vi "SCMP - Externally Triggered Image Acquisition - v2.vi"(0 "FPS":dbl=10.0 format="%.1g", 1 "LCVR Voltages":dbl[][](array[numeric]), 5 "Modulation Cycles":i32=1 min=1 max=30 step=1, 7 "Save to FITS?":bool=TRUE, 9 "Headers In":T12[](array[typedef])=[{"Wavelength (nm)"=530.15, "Exposure (s)"=0.05, "Tuning Delay (ms)"=1000.0, "Beam Type (-1/1)"=1.0, "Tuning Voltages"=[1.111, 2.222, 3.333, 4.444], "Observer"="observer", "Light Shapping Diffuser"=enum."In Beam", "Comment"="", "Data Type"=9, "Mod Cycles"=0, "SCD Calibration Optics"=enum."1 - Polarizer @0, I+Q", "SCD Emission Line Filter"=enum."1-557.6nm", "Cookbook"="", "COMP-S Calibration Wheel"=enum."Dark", "COMP-S Andover Filter Wheel"=enum."530.3nm/HWB 0.34nm (Fe XIV)", "FOV Rotation (deg)"=66.0, "Objective Lens Position (mm)"=0.0, "Occulter size"=0.0, "Time End"=timestamp(3382374145.421875 s since 1904-01-01), "Acc Exposure (s)"=0.0, "Time Stamp Array"=[], "Camera Serial Number"=[], "Camera Temp"=[], "Camera PI (mm)"=[], "Time Start"=timestamp(3382374145.421875 s since 1904-01-01), "Peripherals"={"ILX controler"=FALSE, "Zone temperatures"=FALSE, "Andor"=FALSE, "Andor 2"=FALSE, "PI Stages"=FALSE, "AISAS mechanisms"=FALSE, "AISAS Mech.lvclass"=refnum, "Zone temp ref"=variant, "FWs"=FALSE}, "FITS paths"=[], "Cameras"=enum."Andor", "load preset cbk"=FALSE, "periodic check count"=0, "COMP-S Calibration Wheel 2"=enum."Dark", "Calib"=enum."Dark", "Abso Aperture"=40.0, "Nominal Aperture"=196.0}] {"Nominal Aperture" format="%.1f"; "Abso Aperture" format="%.1f"; "Camera PI (mm)" format="%_3g"; "Acc Exposure (s)" format="%^.3g"; "Occulter size" format="%.2f"; "Objective Lens Position (mm)" min=70.0 max=152.0 format="%.2f"; "FOV Rotation (deg)" format="%.1f"; "Data Type" items=["LIVE", "DARK", "FLAT", "CALI", "OBSE", "ABSO", "AURE", "TARG", "OBJE", "HOLE", "OREX", "THRO", "CHIP"]; "Exposure (s)" format="%^.3g"; "Wavelength (nm)" format="%_6g"}, 11 "error in":errorcluster, 12 "Andor Neo":T13[](array[typedef]) {"Exposure (s)" format="%^.3g"; "Time at Synch" format="%<%H:%M:%S>T"; "Interframe Time" format="%#_3g"; "Frame Readout Time" format="%_3g"; "Row Readout Time" format="%_3g"}) -> (3 "FITS Path Out":path, 6 "Image":u32[][](array[numeric]), 8 "Image Cam2":u32[][](graph), 10 "Headers Out":T2[](array[typedef]) {"Nominal Aperture" format="%.1f"; "Abso Aperture" format="%.1f"; "Camera PI (mm)" format="%_3g"; "Acc Exposure (s)" format="%^.3g"; "Occulter size" format="%.2f"; "Objective Lens Position (mm)" min=70.0 max=152.0 format="%.2f"; "FOV Rotation (deg)" format="%.1f"; "Exposure (s)" format="%^.3g"; "Wavelength (nm)" format="%_6g"}, 13 "FITS Path Out 2":path, 14 "Break":bool, 15 "error out":errorcluster)   [LabVIEW 2014]
doc: "The LL Sequence VI acquires a sequence of images and displays them in an array of image controls using the low-level acquisition VIs. A sequence is appropriate for applications that process multiple images. You can configure a sequence to acquire every frame or to skip a variable number of frames between each image.\n\nTop Level Code Overview\n1) Initialize Camera (Global Shutter, High Well, Low Noise, exposure time, etc.)\n2) Create a buffer set equal in size to the # of trigger pulses (e.g. 100) which is the same as the # of expected images \n3) Start the camera acquisition THEN start the DAQmx task (use merge error cluster to gurantee this)"
uses:
  Camera/Andor Neo Info.ctl
  <vilib>/DAQmx/configure/timing.llb/DAQmx Timing (Use Waveform).vi
  <vilib>/DAQmx/create/channels.llb/DAQmx Create Channel (AO-Voltage-Basic).vi
  <vilib>/DAQmx/write.llb/DAQmx Write (Analog 1D Wfm NChan NSamp).vi
  <vilib>/Waveform/WDTOps.llb/WDT Waveform Duration DBL.vi
  Controls/beaning.ctl
  Controls/SCD - Calibration Optics Filter Wheel.ctl
  AISAS/Controls/Diffuser.ctl
  Controls/SCD - FITS Cluster.ctl
  Controls/SCD - EDT - Emission Line Filter Wheel.ctl
  Controls/CoMP-S Controls/Polarization Optics Filter Wheel.ctl
  Controls/CoMP-S Controls/Emission Line Filter Wheel.ctl
  AISAS/Controls/focus.ctl
  AISAS/Mech/AISAS Mech.lvclass
  Controls/peripherals.ctl
  Controls/Cameras select.ctl
  Controls/FITS Data type.ctl
panel:
  out "mod cycles *4":i32=1
  out "error dequeue":errorcluster
  out "error dequeue 2":errorcluster
  in  "count 2":i32
  in  "Tab Control":T1(tab)
  in  "user break":bool
  out "Image Cam1 Zoom":u32[][](graph)
  out "Image Cam1":u32[][](graph)
  out "# images to acquire":i32
  out "Image Acquisition Started":bool
  out "PixelData [U16]":u16[](array[numeric])
  out "ByteData [U8]":u8[](array[numeric])
  in  "image pointers":u64[](array[numeric])
  in  "imageNo":i32
  in  "count":i32
  out "Acquisition Estimate (s)":dbl format="%0.2f"
  out "# wavelengths":i32=1
  out "Exposure Get (s)":dbl=0.09 format="%_3p"
  out "Image Acq (s)":dbl(slide)=4151.832132564842
  out "# elements in queue":i32
  out "Image Cam":u32[][](graph)
  out "# buffer":i32
  in  "image pointers 2":u64[](array[numeric])
  in  "imageNo 2":i32
  out "# elements in queue 2":i32
  out "# buffer 2":i32
  out "Time Start":timestamp=timestamp(3382374145.421875 s since 1904-01-01) format="%<%H:%M:%S%3u\n%x>T"
  out "Time stamp arr":timestamp[](array[timestamp]) format="%<%H:%M:%S%3u>T"
  out "COMP Waveforms":waveform(dbl)[](graph)
  out "SCD Waveforms":waveform(dbl)[](graph)
  out "Time stamp arr 2":timestamp[](array[timestamp]) format="%<%H:%M:%S%3u>T"
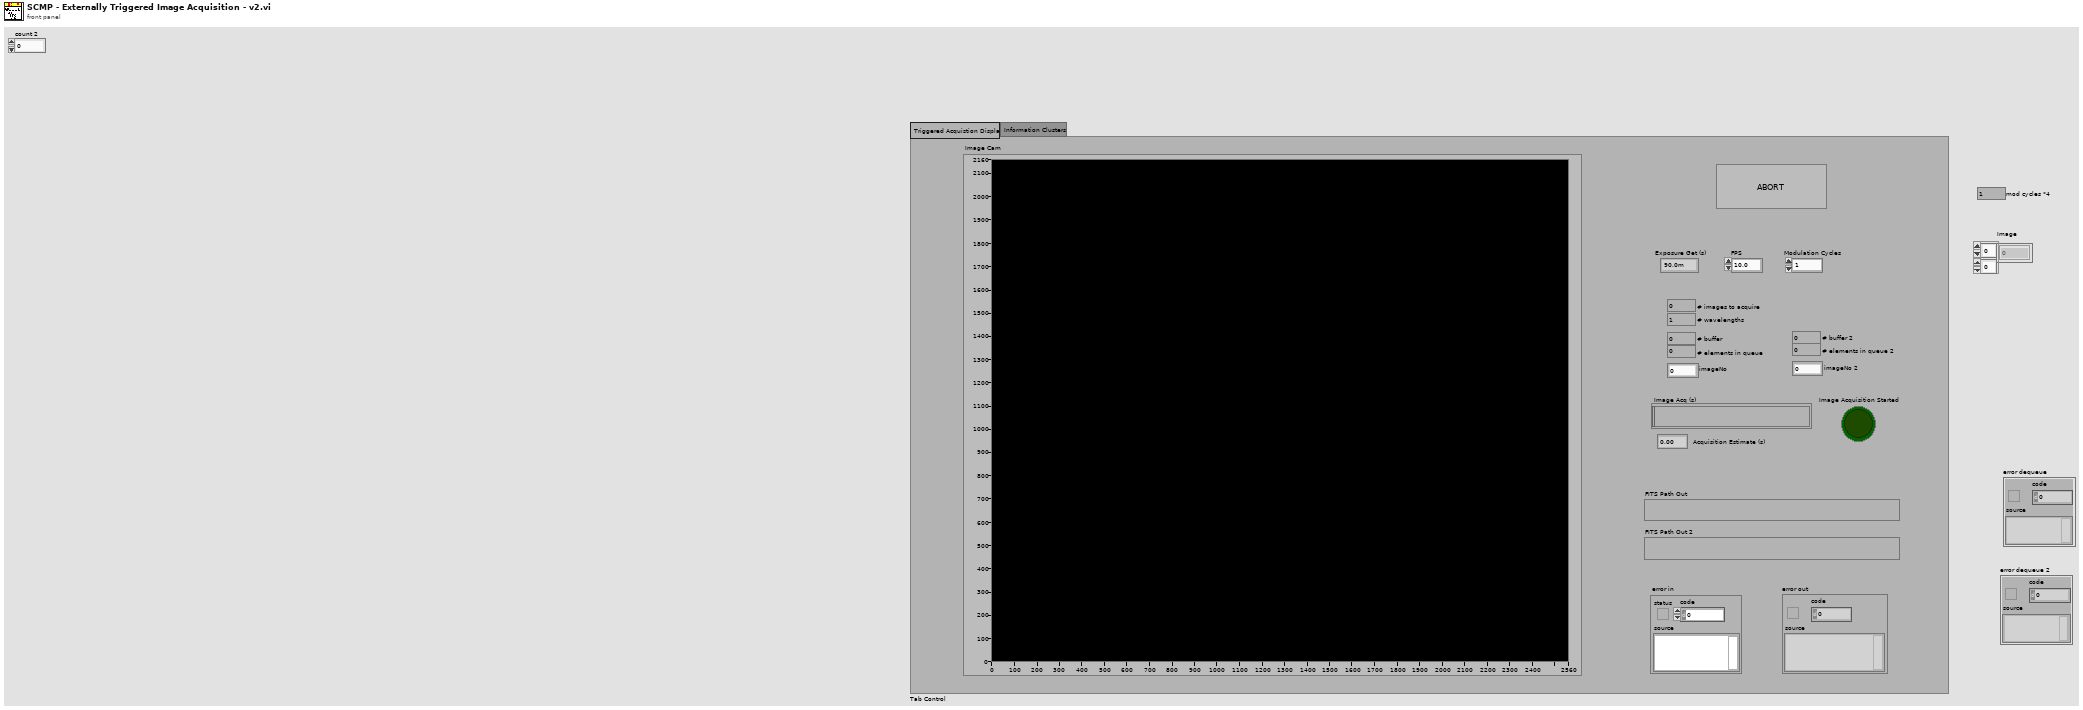
[diagram p1: front panel]
types:
  T1 = enum32{"Triggered Acquistion Display", "Information Clusters"}
  T2 = typedef "SCD - FITS Cluster.ctl" = cluster{"Wavelength (nm)":dbl, "Exposure (s)":dbl, "Tuning Delay (ms)":dbl, "Beam Type (-1/1)":dbl, "Tuning Voltages":dbl[], "Observer":string, "Light Shapping Diffuser":T3, "Comment":string, "Data Type":T4, "Mod Cycles":u16, "SCD Calibration Optics":T5, "SCD Emission Line Filter":T6, "Cookbook":string, "COMP-S Calibration Wheel":T7, "COMP-S Andover Filter Wheel":T8, "FOV Rotation (deg)":dbl, "Objective Lens Position (mm)":T9, "Occulter size":dbl, "Time End":timestamp, "Acc Exposure (s)":dbl, "Time Stamp Array":timestamp[], "Camera Serial Number":string[], "Camera Temp":dbl[], "Camera PI (mm)":dbl[], "Time Start":timestamp, "Peripherals":T10, "FITS paths":path[], "Cameras":T11, "load preset cbk":bool, "periodic check count":i32, "COMP-S Calibration Wheel 2":T7, "Calib":enum16{"Dark", "Flat"}, "Abso Aperture":dbl, "Nominal Aperture":dbl, "Pointer IP":string}
  T3 = typedef "Diffuser.ctl" = enum16{"Out of Beam", "In Beam"}
  T4 = typedef "FITS Data type.ctl" = enum16{"LIVE", "DARK", "FLAT", "CALI", "OBSE", "ABSO", "AURE", "TARG", "OBJE", "HOLE", "OREX", "THRO", "CHIP"}
  T5 = typedef "SCD - Calibration Optics Filter Wheel.ctl" = enum16{"1 - Polarizer @0, I+Q", "2 - Polarizer @90, I-Q", "3 - Polarizer @45, I+U", "4 - Polarizer @135, I-U", "5 - Polarizer @0, Retarder @45, I+V", "6 - Polarizer @0, Retarder @135, I-V", "7 - Dark", "8 - Clear", "9 - N/A"}
  T6 = typedef "SCD - EDT - Emission Line Filter Wheel.ctl" = enum16{"1-557.6nm", "2-587.6nm", "3-589.6nm", "4-630.2nm", "5-656.4nm", "6-849.8nm", "7-854.2nm", "8-866.2nm", "9-1083.0nm"}
  T7 = typedef "Polarization Optics Filter Wheel.ctl" = enum16{"Dark", "Clear", "Exchange Lens", "Polarizer @0, I+Q", "Polarizer @90, I-Q", "Polarizer @45, I+U", "Polarizer @135, I-U", "Polarizer @0, Retarder @45, I+V", "Polarizer @0, Retarder @135, I-V"}
  T8 = typedef "Emission Line Filter Wheel.ctl" = enum16{"530.3nm/HWB 0.34nm (Fe XIV)", "587.6nm/HBW 0.44nm (He I D3)", "637.5nm/HBW 0.53nm (Fe X)", "656.3nm/HBW 0.57nm (H-Alpha)", "789.2nm/HBW 0.85nm (Fe XI)", "854.2nm/HBW 1.01nm (Ca I)", "1074.7nm/HBW 2.34nm (Fe XIII)", "1079.8nm/HBW 1.64nm (Fe XIII)", "1083.0nm/HBW 1.66nm (He I)"}
  T9 = typedef "focus.ctl" = dbl
  T10 = typedef "peripherals.ctl" = cluster{"ILX controler":bool, "Zone temperatures":bool, "Andor":bool, "Andor 2":bool, "PI Stages":bool, "AISAS mechanisms":bool, "AISAS Mech.lvclass":refnum<class "AISAS Mech.lvclass">, "Zone temp ref":variant, "FWs":bool}
  T11 = typedef "Cameras select.ctl" = enum16{"Andor", "GDR"}
  T12 = typedef "SCD - FITS Cluster.ctl" = cluster{"Wavelength (nm)":dbl, "Exposure (s)":dbl, "Tuning Delay (ms)":dbl, "Beam Type (-1/1)":dbl, "Tuning Voltages":dbl[], "Observer":string, "Light Shapping Diffuser":T3, "Comment":string, "Data Type":u16, "Mod Cycles":u16, "SCD Calibration Optics":T5, "SCD Emission Line Filter":T6, "Cookbook":string, "COMP-S Calibration Wheel":T7, "COMP-S Andover Filter Wheel":T8, "FOV Rotation (deg)":dbl, "Objective Lens Position (mm)":T9, "Occulter size":dbl, "Time End":timestamp, "Acc Exposure (s)":dbl, "Time Stamp Array":timestamp[], "Camera Serial Number":string[], "Camera Temp":dbl[], "Camera PI (mm)":dbl[], "Time Start":timestamp, "Peripherals":T10, "FITS paths":path[], "Cameras":T11, "load preset cbk":bool, "periodic check count":i32, "COMP-S Calibration Wheel 2":T7, "Calib":enum16{"Dark", "Flat"}, "Abso Aperture":dbl, "Nominal Aperture":dbl}
  T13 = typedef "Andor Neo Info.ctl" = cluster{"Handle":i32, "Pixel Encoding":string, "AOI Width":i32, "AOI Height":i32, "AOI Stride":i32, "Row Readout Time":dbl, "Frame Readout Time":dbl, "Interframe Time":dbl, "Semaphore":T14, "SerialNumber":string, "Camera Model":string, "Controller ID":string, "Firmware Version":string, "Shutter":string, "BDiv":u8, "Time at Synch":timestamp, "Idx":i32, "PreAmp":string, "Binning":T15, "PixelReadoutRate":string, "Exposure (s)":dbl, "Image Bytes":i64, "Image Pixels":i64, "SpuriousNoiseFilter":bool, "Overlap":bool, "CycleMode":string}
  T14 = typedef "Semaphore RefNum" = refnum<k1>
  T15 = typedef "beaning.ctl" = enum16{"1x1", "2x2", "3x3", "4x4", "8x8"}
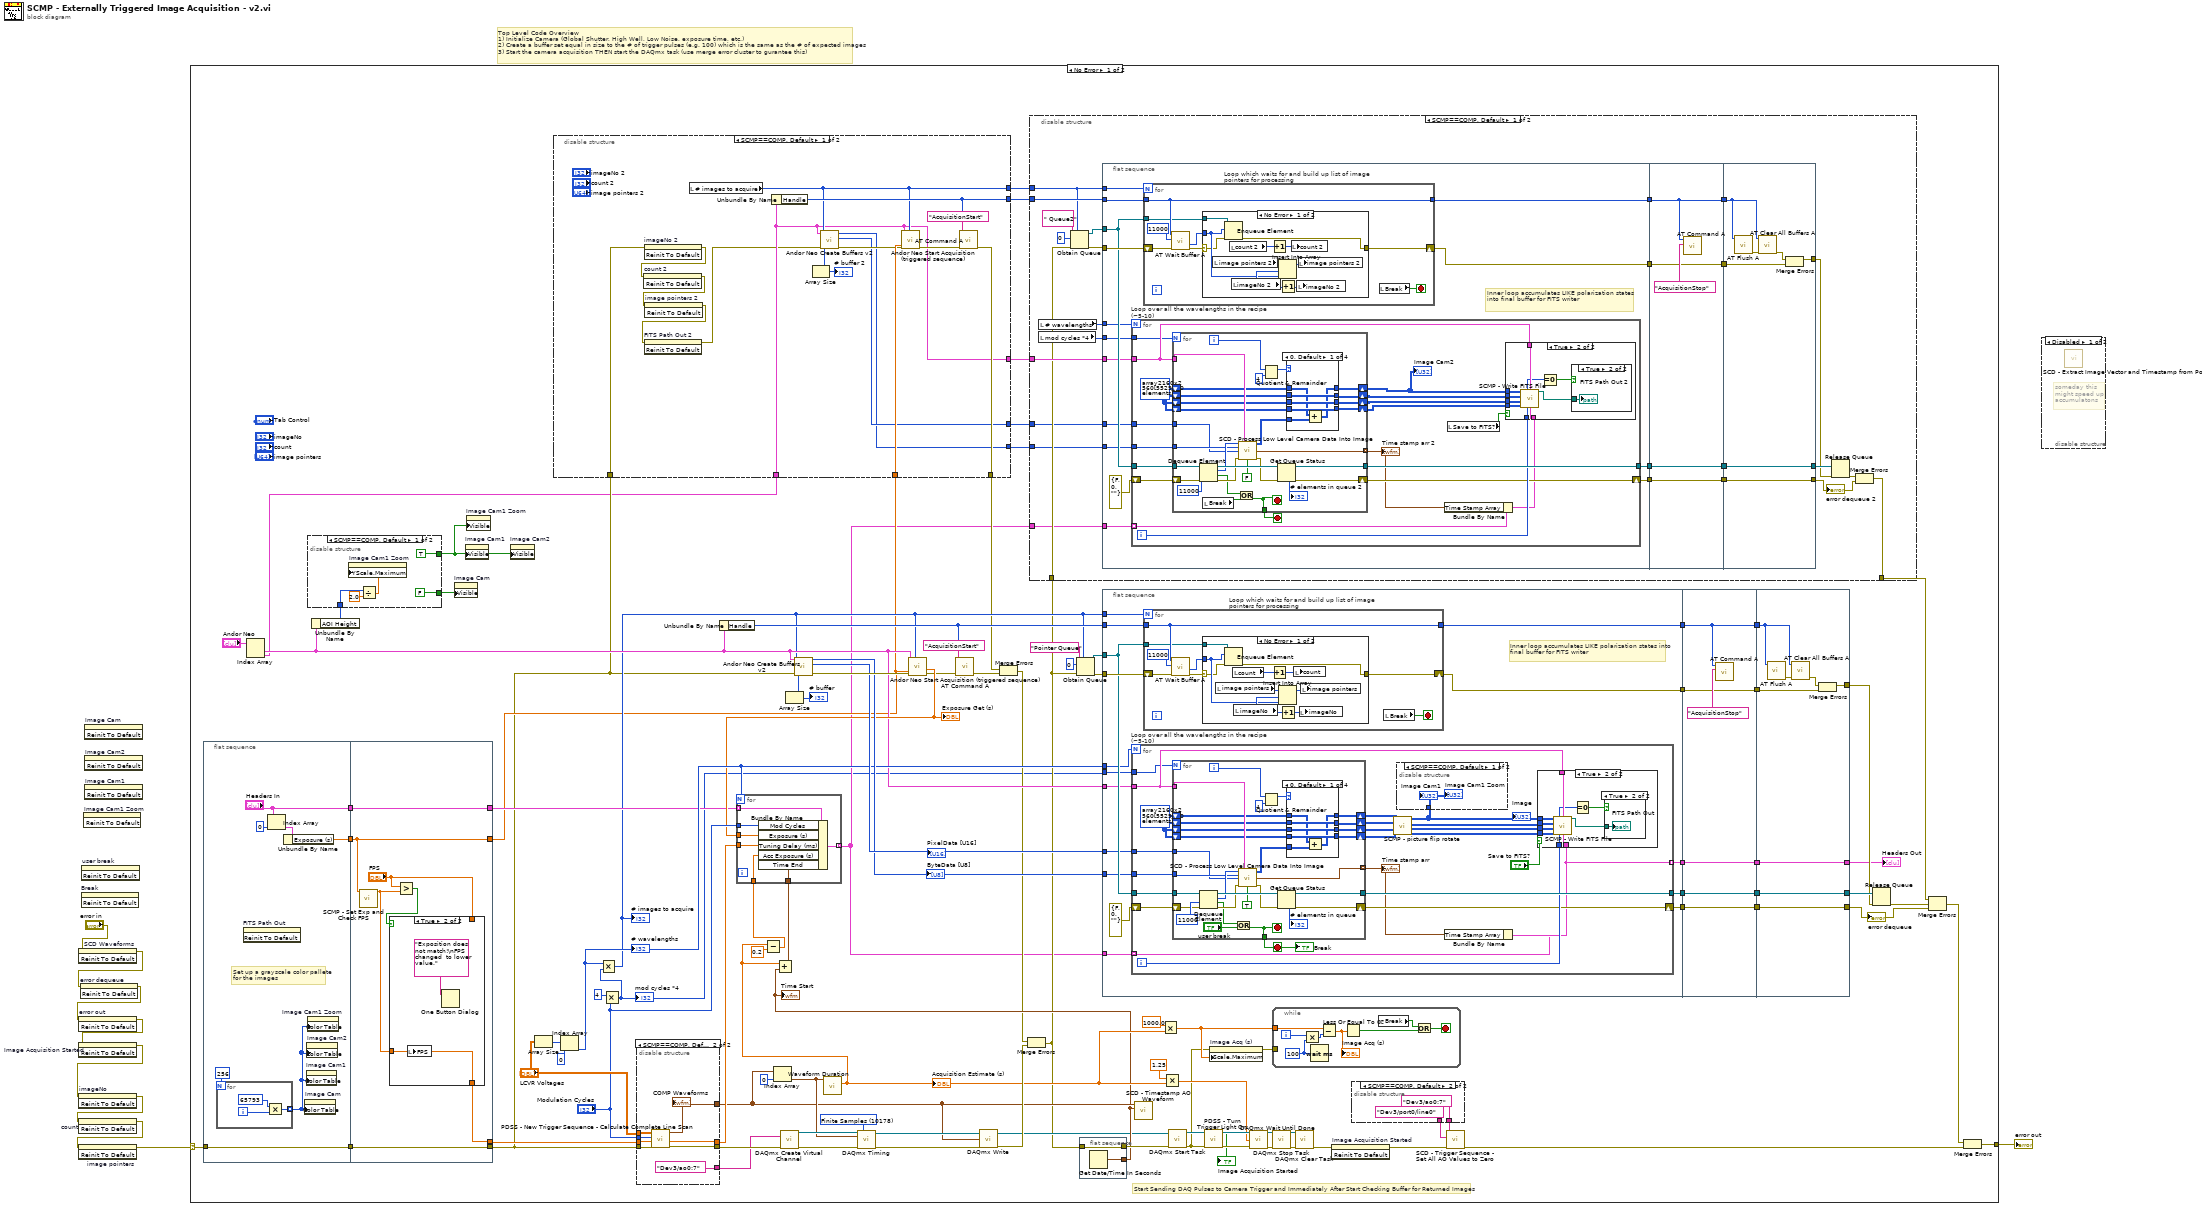
[diagram p0: block diagram]
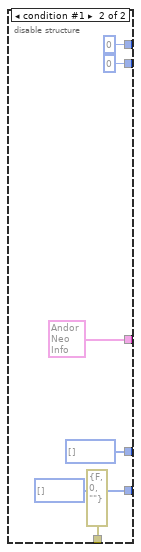
[diagram p3: hidden frame]
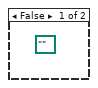
[diagram p4: hidden frame]
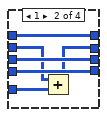
[diagram p6: hidden frame]
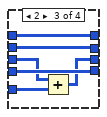
[diagram p7: hidden frame]
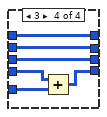
[diagram p8: hidden frame]
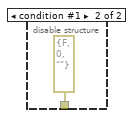
[diagram p10: hidden frame]
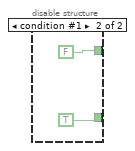
[diagram p12: hidden frame]
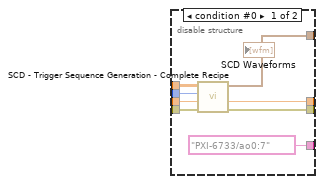
[diagram p13: hidden frame]
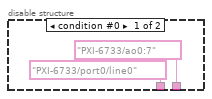
[diagram p14: hidden frame]
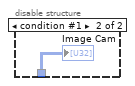
[diagram p15: hidden frame]
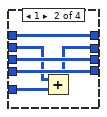
[diagram p18: hidden frame]
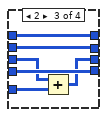
[diagram p19: hidden frame]
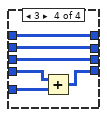
[diagram p20: hidden frame]
diagram:
  # "Top Level Code Overview\n1) Initialize Camera (Global Shutter, High Well, Low Noise, exposure time, etc.)\n2) Create a buffer set equal in size to the # of trigger pulses (e.g. 100) which is the same as the # of expected images \n3) Start the camera acquisition THEN start the DAQmx task (use merge error cluster to gurantee this)"
  n1 = invoke on="SCD Waveforms" class="WFGraph (strict)" method="Reinit To Default"(error in="error in") -> (error out=w3:errorcluster)  [unwired: 2 in, 2 out]
  n2 = invoke on="error dequeue" class="Clust (strict)" method="Reinit To Default"(error in=w3) -> (error out=w2:errorcluster)  [unwired: 2 in, 2 out]
  n3 = invoke on="error out" class="Clust (strict)" method="Reinit To Default"(error in=w2) -> (error out=w8:errorcluster)  [unwired: 2 in, 2 out]
  n4 = invoke on="Image Acquisition Started" class="Bool (strict)" method="Reinit To Default"(error in=w8) -> (error out=w4:errorcluster)  [unwired: 2 in, 2 out]
  n5 = invoke on="imageNo" class="DigNum (strict)" method="Reinit To Default"(error in=w4) -> (error out=w7:errorcluster)  [unwired: 2 in, 2 out]
  n6 = invoke on="count" class="DigNum (strict)" method="Reinit To Default"(error in=w7) -> (error out=w6:errorcluster)  [unwired: 2 in, 2 out]
  n7 = invoke on="image pointers" class="Arr (strict)" method="Reinit To Default"(error in=w6) -> (error out=w5:errorcluster)  [unwired: 2 in, 2 out]
  n8 = invoke on="Break" class="Bool (strict)" method="Reinit To Default"() -> ()  [unwired: 3 in, 3 out]
  n9 = invoke on="user break" class="Bool (strict)" method="Reinit To Default"() -> ()  [unwired: 3 in, 3 out]
  n10 = invoke on="Image Cam1 Zoom" class="IntGraph (strict)" method="Reinit To Default"() -> ()  [unwired: 3 in, 3 out]
  n11 = invoke on="Image Cam" class="IntGraph (strict)" method="Reinit To Default"() -> ()  [unwired: 3 in, 3 out]
  n12 = invoke on="Image Cam2" class="IntGraph (strict)" method="Reinit To Default"() -> ()  [unwired: 3 in, 3 out]
  n13 = invoke on="Image Cam1" class="IntGraph (strict)" method="Reinit To Default"() -> ()  [unwired: 3 in, 3 out]
  n14 = case shown="No Error" w5 {
    selector: w5 -> [w45 w491]
    tunnel: [w82 w491] -> w9
    frame No Error {
      w109 = 10178 items=["Finite Samples"=10178, "Continuous Samples"=10123] ("sample mode")
      # "Start Sending DAQ Pulses to Camera Trigger and Immediately After Start Checking Buffer for Returned Images"
      n15 = flat-sequence {
        tunnel: w45 -> [w294]
        tunnel: [w294] -> w37
        tunnel: ["Headers In"] -> w35
        tunnel: [w289] -> w34
        tunnel: [w305] -> w13
        tunnel: w37 -> [w305]
        tunnel: [w304] -> w36
        tunnel: w35 -> [w304]
        tunnel: [w299] -> w23
        tunnel: w34 -> [w299]
        tunnel: [w302] -> w33
        frame #0 {
          # "Set up a grayscale color pallete for the images"
          n16 = for {
            N: 256 -> [_]
            tunnel: [w297] -> w293 mode=indexing
            i -> [w298]
            n17 = Multiply(x=65793, y=w298) -> (x*y=w297:i32)
          }
          n18 = invoke on="FITS Path Out" class="Path" method="Reinit To Default"() -> ()  [unwired: 3 in, 3 out]
          n19 = Index Array(array="Headers In", index=0) -> (element=w291:T12)
          n20 = Unbundle By Name(w291) -> ("Exposure (s)"=w289:dbl)
          n21 = property on="Image Cam" class="IntGraph (strict)"("Color Table"=w293) -> ()  [unwired: 2 in, 2 out]
          n22 = property on="Image Cam1" class="IntGraph (strict)"("Color Table"=w293) -> ()  [unwired: 2 in, 2 out]
          n23 = property on="Image Cam2" class="IntGraph (strict)"("Color Table"=w293) -> ()  [unwired: 2 in, 2 out]
          n24 = property on="Image Cam1 Zoom" class="IntGraph (strict)"("Color Table"=w293) -> ()  [unwired: 2 in, 2 out]
        }
        frame #1 {
          n25 = call "SCMP - Set Exp and Check FPS.vi"("Exposure [s]"=w299) -> ("FPS"=w300:dbl)  [unwired: 9 in, 1 out]
          n26 = Greater?(x="FPS", y=w300) -> (0:w303:bool)
          n27 = case shown="True" w303 {
            tunnel: [w306 w307] -> w302
            tunnel: "FPS" -> [w306 _]
            tunnel: w300 -> [_ w307]
            frame False {
            }
            frame True {
              n28 = local write "FPS"(w307) -> ()
              n29 = One Button Dialog(message="Exposition does not match!\nFPS changed  to lower value.") -> ()  [unwired: 1 in, 1 out]
            }
          }
        }
      }
      n30 = Index Array(array="Andor Neo") -> (element #1=w27:T13, element #2=w10:T13)  [unwired: 2 in]
      n31 = Unbundle By Name(w27) -> ("AOI Height"=w54:i32)
      n32 = disable-structure shown="SCMP==COMP, Default" {
        disable-tunnel: w54 -> [w312 _]
        disable-tunnel: [TRUE ("Visible") FALSE ("Visible")] -> w46
        disable-tunnel: [FALSE ("Visible") TRUE ("Visible")] -> w53
        frame condition #0 (active) {
          n33 = Divide(x=w312, y=2.0) -> (x/y=w313:dbl)
          n34 = property on="Image Cam1 Zoom" class="IntGraph (strict)"("YScale.Maximum"=w313) -> ()  [unwired: 2 in, 2 out]
        }
        frame condition #1 {
        }
      }
      n35 = property on="Image Cam" class="IntGraph (strict)"("Visible"=w53) -> ()  [unwired: 2 in, 2 out]
      n36 = property on="Image Cam1" class="IntGraph (strict)"("Visible"=w46) -> ()  [unwired: 2 in, 2 out]
      n37 = property on="Image Cam1 Zoom" class="IntGraph (strict)"("Visible"=w46) -> ()  [unwired: 2 in, 2 out]
      n38 = property on="Image Cam2" class="IntGraph (strict)"("Visible"=w46) -> ()  [unwired: 2 in, 2 out]
      n39 = Array Size(array="LCVR Voltages") -> (size(s)=w92:i32[])
      n40 = disable-structure shown="SCMP==COMP, Default" {
        disable-tunnel: w23 -> [w126 _]
        disable-tunnel: [w125 errorcluster {"status"=FALSE, "code"=0, "source"=""} ("error out")] -> w20
        disable-tunnel: [w119 0 ("Handle")] -> w17
        disable-tunnel: [w118 i64[] [] ("PixelData")] -> w16
        disable-tunnel: [w117 u8[] [] ("ByteData")] -> w15
        disable-tunnel: [w116 0 ("# images to acquire")] -> w14
        disable-tunnel: w13 -> [w112 _]
        disable-tunnel: [w115 T13 {"Handle"=0, "Pixel Encoding"="", "AOI Width"=0, "AOI Height"=0, "AOI Stride"=0, "Row Readout Time"=0.0, "Frame Readout Time"=0.0, "Interframe Time"=0.0, "Semaphore"=refnum, "SerialNumber"="", "Camera Model"="", "Controller ID"="", "Firmware Version"="", "Shutter"="Global", "BDiv"=1, "Time at Synch"=timestamp(3029526000.379448 s since 1904-01-01), "Idx"=0, "PreAmp"="", "Binning"=enum."1x1", "PixelReadoutRate"="", "Exposure (s)"=0.05, "Image Bytes"=0, "Image Pixels"=0, "SpuriousNoiseFilter"=FALSE, "Overlap"=FALSE, "CycleMode"=""} ("Neo Info")] -> w11
        disable-tunnel: w10 -> [w115 _]
        frame condition #0 (active) {
          n41 = invoke on="imageNo 2" class="DigNum (strict)" method="Reinit To Default"(error in=w112) -> (error out=w114:errorcluster)  [unwired: 2 in, 2 out]
          n42 = invoke on="count 2" class="DigNum (strict)" method="Reinit To Default"(error in=w114) -> (error out=w113:errorcluster)  [unwired: 2 in, 2 out]
          n43 = invoke on="image pointers 2" class="Arr (strict)" method="Reinit To Default"(error in=w113) -> (error out=w111:errorcluster)  [unwired: 2 in, 2 out]
          n44 = invoke on="FITS Path Out 2" class="Path" method="Reinit To Default"(error in=w111) -> (error out=w110:errorcluster)  [unwired: 2 in, 2 out]
          n45 = local read "# images to acquire"() -> (w116:i32)
          n46 = Unbundle By Name(w115) -> ("Handle"=w119:i32)
          n47 = call "Andor Neo Create Buffers v2.vi"("error in"=w110, "Number of Images"=w116, "Camera Info"=w115) -> ("error out"=w123:errorcluster, "PixelData"=w118:i64[], "ByteData"=w117:u8[], "# of Andor buffers"=w121:i32)  [unwired: 4 in, 1 out]
          n48 = Array Size(array=w121) -> (size(s)=→"# buffer 2":i32)
          n49 = call "Andor Neo Start Acquisition (triggered sequence).vi"("Exposure Set (s)"=w126, "error in"=w123, "Frames"=w116, "Camera Info"=w115) -> ("error out"=w122:errorcluster)  [unwired: 6 in, 1 out]
          n50 = call <userlib>:"AT Command A.vi"("error in (no error)"=w122, "Feature"="AcquisitionStart" ("Command"), "Handle"=w119) -> ("error out"=w125:errorcluster)  [unwired: 7 in, 1 out]
        }
        frame condition #1 {
        }
      }
      n51 = Index Array(array=w92, index=0) -> (element=w55:i32)
      "# wavelengths" <- w55
      n52 = Multiply(x=4 ("value"), y="Modulation Cycles") -> (x*y=w12:i32)
      "mod cycles *4" <- w12
      n53 = Multiply(x=w55, y=w12) -> (x*y=w24:i32)
      "# images to acquire" <- w24
      n54 = disable-structure shown="SCMP==COMP, Default" {
        disable-tunnel: [w323 w327] -> w100
        disable-tunnel: "LCVR Voltages" -> [w322 w331]
        disable-tunnel: [w317 w325] -> w60
        disable-tunnel: w33 -> [w321 w329]
        disable-tunnel: w13 -> [w320 w328]
        disable-tunnel: [w319 w326] -> w63
        disable-tunnel: "Modulation Cycles" -> [w318 w330]
        disable-tunnel: [tag "PXI-6733/ao0:7" ("physical channels") tag "Dev3/ao0:7" ("physical channels")] -> w31
        frame condition #0 {
          n55 = call "SCD - Trigger Sequence Generation - Complete Recipe.vi"("error in"=w320, "FPS"=w321, "Modulation Cycles\nAt Each Wavelength"=w318, "LCVR Voltages"=w322) -> ("error out"=w323:errorcluster, "LCVR Relaxtion Time"=w319:dbl, "SCD Waveforms (Graph)"=w317:waveform(dbl)[])  [unwired: 5 in]
          "SCD Waveforms" <- w317
        }
        frame condition #1 (active) {
          n56 = call "PDSS - New Trigger Sequence - Calculate Complete Line Scan.vi"("error in"=w328, "FPS"=w329, "Modulation Cycles\nAt Each Wavelength"=w330, "LCVR Voltages"=w331) -> ("error out"=w327:errorcluster, "LCVR Relaxtion Time"=w326:dbl, "AO Graph"=w325:waveform(dbl)[])  [unwired: 5 in]
          "COMP Waveforms" <- w325
        }
      }
      n57 = Unbundle By Name(w27) -> ("Handle"=w26:i32)
      n58 = Index Array(array=w60, index=0) -> (element=w97:waveform(dbl))
      n59 = call-poly <vilib>:"DAQmx Create Virtual Channel.vi"("physical channels"=w31, "error in"=w100) -> ("task out"=w107:refnum<k21>, "error out"=w108:errorcluster)  [unwired: 12 in]
      n60 = call "Andor Neo Create Buffers v2.vi"("error in"=w13, "Number of Images"=w24, "Camera Info"=w27) -> ("error out"=w81:errorcluster, "PixelData"=w77:i64[], "ByteData"=w76:u8[], "# of Andor buffers"=w44:i32)  [unwired: 4 in, 1 out]
      "ByteData [U8]" <- w76
      "PixelData [U16]" <- w77
      n61 = Array Size(array=w44) -> (size(s)=→"# buffer":i32)
      n62 = call-poly <vilib>:"Waveform Duration.vi"("waveform in"=w97) -> ("duration"=w48:dbl)  [unwired: 8 in, 2 out]
      "Acquisition Estimate (s)" <- w48
      n63 = Subtract(x=w48, y=0.2) -> (x-y=w47:dbl)
      n64 = Add(x=w48, y=w32) -> (x+y=w52:timestamp)
      n65 = call-poly <vilib>:"DAQmx Timing.vi"("task/channels in"=w107, "sample mode"=w109, "waveform"=w97, "error in"=w108) -> ("task out"=w98:refnum<k21>, "error out"=w99:errorcluster)  [unwired: 10 in]
      n66 = call "Andor Neo Start Acquisition (triggered sequence).vi"("Exposure Set (s)"=w23, "error in"=w81, "Frames"=w24, "Camera Info"=w27) -> ("error out"=w50:errorcluster, "Exposure Get (s)"=w51:dbl)  [unwired: 6 in]
      "Exposure Get (s)" <- w51
      n67 = for {
        N: w55 -> [_]
        tunnel: [w350] -> w19 mode=indexing
        tunnel: w51 -> [w349]
        tunnel: w36 -> [w348] mode=indexing
        tunnel: w63 -> [w347]
        tunnel: "Modulation Cycles" -> [w346]
        tunnel: w47 -> [w345]
        tunnel: w52 -> [w344]
        n68 = Bundle By Name(cluster=w348, "Mod Cycles"=w346, "Exposure (s)"=w349, "Tuning Delay (ms)"=w347, "Acc Exposure (s)"=w345, "Time End"=w344) -> (w350:T12)
      }
      n69 = call <userlib>:"AT Command A.vi"("error in (no error)"=w50, "Feature"="AcquisitionStart" ("Command"), "Handle"=w26) -> ("error out"=w80:errorcluster)  [unwired: 7 in, 1 out]
      n70 = call-poly <vilib>:"DAQmx Write.vi"("task/channels in"=w98, "data"=w60, "error in"=w99) -> ("task out"=w25:refnum<k21>, "error out"=w84:errorcluster)  [unwired: 10 in, 1 out]
      n71 = Merge Errors(w20, w80) -> (w21:errorcluster)
      n72 = Merge Errors(w21, w84) -> (w22:errorcluster)
      n73 = disable-structure shown="SCMP==COMP, Default" {
        disable-tunnel: w11 -> [w150 _]
        disable-tunnel: w22 -> [w149 _]
        disable-tunnel: w19 -> [w148 _]
        disable-tunnel: [w147 errorcluster {"status"=FALSE, "code"=0, "source"=""} ("error IO")] -> w18
        disable-tunnel: w17 -> [w144 _]
        disable-tunnel: w16 -> [w143 _]
        disable-tunnel: w15 -> [w142 _]
        disable-tunnel: w14 -> [w139 _]
        frame condition #0 (active) {
          n74 = local read "# wavelengths"() -> (w138:i32)
          n75 = local read "mod cycles *4"() -> (w133:i32)
          n76 = Obtain Queue(max queue size (-1, unlimited)=w139, name (unnamed)=" Queue2", element data type=u64 0 ("Output buffer"), error in (no error)=w149) -> (queue out=w141:refnum<queue>, error out=w140:errorcluster)  [unwired: 1 in, 1 out]
          n77 = flat-sequence {
            tunnel: w140 -> [w173]
            tunnel: w144 -> [w172]
            tunnel: [w171] -> w158
            tunnel: [w162] -> w157
            tunnel: w150 -> [w166]
            tunnel: w143 -> [w167]
            tunnel: w142 -> [w169]
            tunnel: w141 -> [w170]
            tunnel: [w168] -> w156
            tunnel: w133 -> [w164]
            tunnel: [w165] -> w155
            tunnel: w139 -> [w161]
            tunnel: w148 -> [w160]
            tunnel: w138 -> [w159]
            tunnel: w158 -> [w277]
            tunnel: w157 -> [w276]
            tunnel: w156 -> [w279]
            tunnel: w155 -> [w278]
            tunnel: [w277] -> w154
            tunnel: [w279] -> w153
            tunnel: [w278] -> w152
            tunnel: [w276] -> w151
            tunnel: [w287] -> w135
            tunnel: [w286] -> w134
            tunnel: w154 -> [w284]
            tunnel: w153 -> [w282]
            tunnel: w152 -> [w287]
            tunnel: w151 -> [w285]
            tunnel: [w282] -> w136
            frame #0 {
              # "Inner loop accumulates LIKE polarization states into final buffer for FITS writer"
              n78 = for "Loop over all the wavelengths in the recipe (~5-10)" {
                N: w159 -> [_]
                tunnel: w170 -> [w192]
                tunnel: w169 -> [w191]
                tunnel: [w190] -> w168
                tunnel: w167 -> [w189]
                tunnel: w166 -> [w187]
                tunnel: w164 -> [w186]
                shift-right: [w184] -> w165
                shift-left: errorcluster {"status"=FALSE, "code"=0, "source"=""} ("error out") -> [w183]
                tunnel: w160 -> [w179] mode=indexing
                i -> [w185]
                stop <- w182 stop-if-true
                w188 = u32[][] array2160x2560[5529600 elements] ("2560x2160 Initialized Array")
                n79 = for {
                  N: w186 -> [_]
                  tunnel: w192 -> [w232]
                  tunnel: w191 -> [w229]
                  tunnel: [w215] -> w190
                  tunnel: w189 -> [w228]
                  tunnel: w187 -> [w227]
                  shift-right: [w220] -> w177
                  shift-left: w188 -> [w221]
                  shift-right: [w219] -> w176
                  shift-left: w188 -> [w222]
                  shift-right: [w218] -> w175
                  shift-left: w188 -> [w223]
                  shift-right: [w217] -> w174
                  shift-left: w188 -> [w224]
                  shift-right: [w210] -> w184
                  shift-left: w183 -> [w208]
                  tunnel: [w205] -> w182
                  tunnel: [w207] -> w180 mode=indexing
                  i -> [w209]
                  stop <- w205 stop-if-true
                  n80 = Dequeue Element(queue=w232, timeout in ms (-1)=11000, error in (no error)=w208) -> (queue out=w231:refnum<queue>, element=w230:u64, timed out?=w204:bool, error out=w212:errorcluster)
                  n81 = local read "Break"() -> (w203:bool)
                  n82 = Or(x=w204, y=w203) -> (x .or. y?=w205:bool)
                  n83 = call "SCD - Process Low Level Camera Data Into Image.vi"("Pointer In"=w230, "Neo Info"=w227, "ByteData (U8)"=w229, "PixelData (U16)"=w228, "error in (no error)"=w212, "scmp demo pic"=FALSE) -> ("Image (I32)"=w216:u32[][], "Timestamp"=w207:timestamp, "error out"=w211:errorcluster)  [unwired: 7 in]
                  n84 = Quotient & Remainder(x=w209, y=4) -> (x-y*floor(x/y)=w225:i32)  [unwired: 1 out]
                  n85 = Get Queue Status(queue=w231, error in (no error)=w211) -> (queue out=w215:refnum<queue>, error out=w210:errorcluster, # elements in queue=→"# elements in queue 2":i32)  [unwired: 1 in, 5 out]
                  n86 = case shown="0, Default" w225 {
                    tunnel: w224 -> [w236 w243 w249 w252]
                    tunnel: w223 -> [w237 w244 w246 w255]
                    tunnel: w222 -> [w238 w240 w250 w256]
                    tunnel: w221 -> [w234 w241 w247 w253]
                    tunnel: [w233 w241 w247 w253] -> w220
                    tunnel: [w238 w239 w250 w256] -> w219
                    tunnel: [w237 w244 w245 w255] -> w218
                    tunnel: [w236 w243 w249 w251] -> w217
                    tunnel: w216 -> [w235 w242 w248 w254]
                    frame 0, Default {
                      n87 = Add(x=w234, y=w235) -> (x+y=w233:u32[][])
                    }
                    frame 1 {
                      n88 = Add(x=w240, y=w242) -> (x+y=w239:u32[][])
                    }
                    frame 2 {
                      n89 = Add(x=w246, y=w248) -> (x+y=w245:u32[][])
                    }
                    frame 3 {
                      n90 = Add(x=w252, y=w254) -> (x+y=w251:u32[][])
                    }
                  }
                }
                "Time stamp arr 2" <- w180
                "Image Cam2" <- w177
                n91 = Bundle By Name(cluster=w179, "Time Stamp Array"=w180) -> (w181:T12)
                n92 = local read "Save to FITS?"() -> (w178:bool)
                n93 = case shown="True" w178 {
                  tunnel: w176 -> [_ w199]
                  tunnel: w175 -> [_ w200]
                  tunnel: w174 -> [_ w201]
                  tunnel: w181 -> [_ w197]
                  tunnel: w177 -> [_ w198]
                  tunnel: w187 -> [_ w196]
                  tunnel: w185 -> [_ w195]
                  frame False {
                    (unwired) path "" ("FITS Path Out")
                  }
                  frame True {
                    n94 = call "SCMP - Write FITS File.vi"("A"=w198, "FITS Header"=w197, "Neo Info"=w196, "B"=w199, "C"=w200, "D"=w201, "Image #"=w195) -> ("FITS Path Out"=w194:path)  [unwired: 6 in, 2 out]
                    n95 = Equal To 0?(x=w195) -> (x = 0?=w193:bool)
                    n96 = case shown="True" w193 {
                      tunnel: w194 -> [_ w202]
                      frame False {
                      }
                      frame True {
                        "FITS Path Out 2" <- w202
                      }
                    }
                  }
                }
              }
              n97 = for "Loop which waits for and build up list of image pointers for processing" {
                N: w161 -> [_]
                tunnel: w172 -> [w261]
                tunnel: [w261] -> w171
                tunnel: w170 -> [w259]
                shift-right: [w258] -> w162
                shift-left: w173 -> [w263]
                stop <- w257 stop-if-true
                n98 = call <userlib>:"AT Wait Buffer A.vi"("error in (no error)"=w263, "Timeout"=u32 11000, "Handle"=w261) -> ("error out"=w260:errorcluster, "Output buffer"=w262:u64)  [unwired: 5 in, 2 out]
                n99 = case shown="No Error" w260 {
                  selector: w260 -> [w266 w275]
                  tunnel: w262 -> [w268 _]
                  tunnel: [w265 w275] -> w258
                  tunnel: w259 -> [w267 _]
                  frame No Error {
                    n100 = local read "image pointers 2"() -> (w272:u64[])
                    n101 = Enqueue Element(queue=w267, element=w268, error in (no error)=w266) -> (error out=w265:errorcluster)  [unwired: 1 in, 2 out]
                    n102 = local read "count 2"() -> (w274:i32)
                    n103 = local read "imageNo 2"() -> (w269:i32)
                    n104 = Increment(x=w274) -> (x+1=w273:i32)
                    n105 = Insert Into Array(array=w272, index=w269, new element=w268) -> (w271:u64[])
                    n106 = Increment(x=w269) -> (x+1=w270:i32)
                    n107 = local write "count 2"(w273) -> ()
                    n108 = local write "imageNo 2"(w270) -> ()
                    n109 = local write "image pointers 2"(w271) -> ()
                  }
                  frame Error {
                  }
                }
                n110 = local read "Break"() -> (w257:bool)
              }
            }
            frame #1 {
              n111 = call <userlib>:"AT Command A.vi"("Feature"="AcquisitionStop" ("Command"), "Handle"=w277) -> ()  [unwired: 8 in, 2 out]
            }
            frame #2 {
              n112 = call <userlib>:"AT Flush A.vi"("Handle"=w284) -> ("error out"=w281:errorcluster)  [unwired: 9 in, 1 out]
              n113 = call <userlib>:"AT Clear All Buffers A.vi"("error in (no error)"=w281, "Handle"=w284) -> ("error out"=w283:errorcluster)  [unwired: 8 in, 1 out]
              n114 = Merge Errors(w283, w285) -> (w286:errorcluster)
            }
          }
          n115 = Release Queue(queue=w136, error in (no error)=w134) -> (error out=w137:errorcluster)  [unwired: 1 in, 2 out]
          n116 = Merge Errors(w137, w135) -> (w147:errorcluster)
          "error dequeue 2" <- w135
        }
        frame condition #1 {
        }
      }
      n117 = Obtain Queue(max queue size (-1, unlimited)=w24, name (unnamed)="Pointer Queue", element data type=u64 0 ("Output buffer"), error in (no error)=w22) -> (queue out=w73:refnum<queue>, error out=w74:errorcluster)  [unwired: 1 in, 1 out]
      n118 = flat-sequence {
        tunnel: [w352] -> w79
        tunnel: w22 -> [w352]
        tunnel: [w351] -> w32
        frame #0 {
          n119 = Get Date/Time In Seconds() -> (seconds since 1Jan1904=w351:timestamp)
        }
      }
      n120 = flat-sequence {
        tunnel: w74 -> [w368]
        tunnel: w24 -> [w358]
        tunnel: w26 -> [w367]
        tunnel: [w366] -> w86
        tunnel: [w353] -> w85
        tunnel: w27 -> [w359]
        tunnel: w19 -> [w361]
        tunnel: [w360] -> w78
        tunnel: w77 -> [w362]
        tunnel: w76 -> [w364]
        tunnel: w73 -> [w365]
        tunnel: [w363] -> w71
        tunnel: w55 -> [w356]
        tunnel: w12 -> [w355]
        tunnel: [w357] -> w58
        tunnel: w86 -> [w478]
        tunnel: w85 -> [w477]
        tunnel: w78 -> [w481]
        tunnel: w71 -> [w480]
        tunnel: w58 -> [w479]
        tunnel: [w478] -> w42
        tunnel: [w481] -> w41
        tunnel: [w480] -> w40
        tunnel: [w479] -> w39
        tunnel: [w477] -> w38
        tunnel: [w488] -> w29
        tunnel: [w489] -> w70
        tunnel: [w490] -> w66
        tunnel: [w487] -> w67
        tunnel: w42 -> [w485]
        tunnel: w41 -> [w490]
        tunnel: w40 -> [w489]
        tunnel: w39 -> [w488]
        tunnel: w38 -> [w486]
        frame #0 {
          # "Inner loop accumulates LIKE polarization states into final buffer for FITS writer"
          n121 = for "Loop over all the wavelengths in the recipe (~5-10)" {
            N: w356 -> [_]
            tunnel: w365 -> [w391]
            tunnel: w364 -> [w390]
            tunnel: [w389] -> w363
            tunnel: w362 -> [w388]
            tunnel: w361 -> [w370] mode=indexing
            tunnel: [w371] -> w360 mode=indexing
            tunnel: w359 -> [w386]
            tunnel: w355 -> [w385]
            shift-right: [w382] -> w357
            shift-left: errorcluster {"status"=FALSE, "code"=0, "source"=""} ("error out") -> [w373]
            i -> [w384]
            stop <- w372 stop-if-true
            w387 = u32[][] array2160x2560[5529600 elements] ("2560x2160 Initialized Array")
            n122 = for {
              N: w385 -> [_]
              tunnel: w391 -> [w433]
              tunnel: w390 -> [w430]
              tunnel: [w416] -> w389
              tunnel: w388 -> [w429]
              tunnel: w386 -> [w428]
              shift-right: [w421] -> w381
              shift-left: w387 -> [w422]
              shift-right: [w420] -> w380
              shift-left: w387 -> [w423]
              shift-right: [w419] -> w379
              shift-left: w387 -> [w424]
              shift-right: [w418] -> w378
              shift-left: w387 -> [w425]
              shift-right: [w411] -> w382
              shift-left: w373 -> [w409]
              tunnel: [w406] -> w372
              tunnel: [w408] -> w369 mode=indexing
              i -> [w410]
              stop <- w406 stop-if-true
              n123 = Dequeue Element(queue=w433, timeout in ms (-1)=11000, error in (no error)=w409) -> (queue out=w432:refnum<queue>, element=w431:u64, timed out?=w405:bool, error out=w413:errorcluster)
              n124 = Or(x=w405, y="user break") -> (x .or. y?=w406:bool)
              n125 = call "SCD - Process Low Level Camera Data Into Image.vi"("Pointer In"=w431, "Neo Info"=w428, "ByteData (U8)"=w430, "PixelData (U16)"=w429, "error in (no error)"=w413, "scmp demo pic"=TRUE) -> ("Image (I32)"=w417:u32[][], "Timestamp"=w408:timestamp, "error out"=w412:errorcluster)  [unwired: 7 in]
              n126 = Quotient & Remainder(x=w410, y=4) -> (x-y*floor(x/y)=w426:i32)  [unwired: 1 out]
              n127 = Get Queue Status(queue=w432, error in (no error)=w412) -> (queue out=w416:refnum<queue>, error out=w411:errorcluster, # elements in queue=→"# elements in queue":i32)  [unwired: 1 in, 5 out]
              n128 = case shown="0, Default" w426 {
                tunnel: w425 -> [w437 w444 w450 w453]
                tunnel: w424 -> [w438 w445 w447 w456]
                tunnel: w423 -> [w439 w441 w451 w457]
                tunnel: w422 -> [w435 w442 w448 w454]
                tunnel: [w434 w442 w448 w454] -> w421
                tunnel: [w439 w440 w451 w457] -> w420
                tunnel: [w438 w445 w446 w456] -> w419
                tunnel: [w437 w444 w450 w452] -> w418
                tunnel: w417 -> [w436 w443 w449 w455]
                frame 0, Default {
                  n129 = Add(x=w435, y=w436) -> (x+y=w434:u32[][])
                }
                frame 1 {
                  n130 = Add(x=w441, y=w443) -> (x+y=w440:u32[][])
                }
                frame 2 {
                  n131 = Add(x=w447, y=w449) -> (x+y=w446:u32[][])
                }
                frame 3 {
                  n132 = Add(x=w453, y=w455) -> (x+y=w452:u32[][])
                }
              }
            }
            "Time stamp arr" <- w369
            "Break" <- w372
            n133 = call "SCMP - picture flip rotate.vi"("D"=w378, "C"=w379, "B"=w380, "A"=w381) -> ("Array D"=w375:u32[][], "Array C"=w376:u32[][], "Array B"=w377:u32[][], "Array A"=w374:u32[][])  [unwired: 4 in]
            "Image" <- w374
            n134 = disable-structure shown="SCMP==COMP, Default" {
              disable-tunnel: w374 -> [w392 w393]
              frame condition #0 (active) {
                "Image Cam1" <- w392
                "Image Cam1 Zoom" <- w392
              }
              frame condition #1 {
                "Image Cam" <- w393
              }
            }
            n135 = Bundle By Name(cluster=w370, "Time Stamp Array"=w369) -> (w371:T12)
            n136 = case shown="True" "Save to FITS?" {
              tunnel: w377 -> [_ w400]
              tunnel: w376 -> [_ w401]
              tunnel: w375 -> [_ w402]
              tunnel: w371 -> [_ w398]
              tunnel: w374 -> [_ w399]
              tunnel: w386 -> [_ w397]
              tunnel: w384 -> [_ w396]
              frame False {
              }
              frame True {
                n137 = call "SCMP - Write FITS File.vi"("A"=w399, "FITS Header"=w398, "Neo Info"=w397, "B"=w400, "C"=w401, "D"=w402, "Image #"=w396) -> ("FITS Path Out"=w394:path)  [unwired: 6 in, 2 out]
                n138 = Equal To 0?(x=w396) -> (x = 0?=w395:bool)
                n139 = case shown="True" w395 {
                  tunnel: w394 -> [_ w403]
                  frame False {
                  }
                  frame True {
                    "FITS Path Out" <- w403
                  }
                }
              }
            }
          }
          n140 = for "Loop which waits for and build up list of image pointers for processing" {
            N: w358 -> [_]
            tunnel: w367 -> [w462]
            tunnel: [w462] -> w366
            tunnel: w365 -> [w460]
            shift-right: [w459] -> w353
            shift-left: w368 -> [w464]
            stop <- w458 stop-if-true
            n141 = call <userlib>:"AT Wait Buffer A.vi"("error in (no error)"=w464, "Timeout"=u32 11000, "Handle"=w462) -> ("error out"=w461:errorcluster, "Output buffer"=w463:u64)  [unwired: 5 in, 2 out]
            n142 = case shown="No Error" w461 {
              selector: w461 -> [w467 w476]
              tunnel: w463 -> [w469 _]
              tunnel: [w466 w476] -> w459
              tunnel: w460 -> [w468 _]
              frame No Error {
                n143 = local read "image pointers"() -> (w473:u64[])
                n144 = Enqueue Element(queue=w468, element=w469, error in (no error)=w467) -> (error out=w466:errorcluster)  [unwired: 1 in, 2 out]
                n145 = local read "count"() -> (w475:i32)
                n146 = local read "imageNo"() -> (w470:i32)
                n147 = Increment(x=w475) -> (x+1=w474:i32)
                n148 = Insert Into Array(array=w473, index=w470, new element=w469) -> (w472:u64[])
                n149 = Increment(x=w470) -> (x+1=w471:i32)
                n150 = local write "count"(w474) -> ()
                n151 = local write "imageNo"(w471) -> ()
                n152 = local write "image pointers"(w472) -> ()
              }
              frame Error {
              }
            }
            n153 = local read "Break"() -> (w458:bool)
          }
        }
        frame #1 {
          n154 = call <userlib>:"AT Command A.vi"("Feature"="AcquisitionStop" ("Command"), "Handle"=w478) -> ()  [unwired: 8 in, 2 out]
        }
        frame #2 {
          n155 = call <userlib>:"AT Flush A.vi"("Handle"=w485) -> ("error out"=w483:errorcluster)  [unwired: 9 in, 1 out]
          n156 = call <userlib>:"AT Clear All Buffers A.vi"("error in (no error)"=w483, "Handle"=w485) -> ("error out"=w484:errorcluster)  [unwired: 8 in, 1 out]
          n157 = Merge Errors(w484, w486) -> (w487:errorcluster)
        }
      }
      n158 = call "SCD - Timestamp AO Waveform.vi"("DAQ To"=w32, "SCD AO Waveforms"=w60) -> ()  [unwired: 8 in, 2 out]
      n159 = Multiply(x=1000.0, y=w48) -> (x*y=w68:dbl)
      n160 = Multiply(x=1.25, y=w48) -> (x*y=w88:dbl)
      n161 = call <vilib>:"DAQmx Start Task.vi"("task/channels in"=w25, "error in"=w79) -> ("task out"=w106:refnum<k21>, "error out"=w65:errorcluster)  [unwired: 12 in]
      n162 = call "PDSS - Turn Trigger Light On.vi"("error in (no error)"=w65) -> ("error out"=w95:errorcluster, "Trigger Started"=→"Image Acquisition Started":bool)  [unwired: 9 in]
      n163 = property on="Image Acq (s)" class="Slide (strict)"(error in=w65, "Scale.Maximum"=w68) -> (error out=w64:errorcluster)  [unwired: 1 in, 1 out]
      n164 = call <vilib>:"DAQmx Wait Until Done.vi"("task/channels in"=w106, "timeout (sec)"=w88, "error in"=w95) -> ("task out"=w105:refnum<k21>, "error out"=w104:errorcluster)  [unwired: 11 in]
      n165 = while {
        tunnel: w68 -> [w342]
        tunnel: w64 -> [_]
        i -> [w340]
        stop <- w337 stop-if-true
        w339 = u32 100 ("milliseconds to wait")
        n166 = Multiply(x=w340, y=w339) -> (x*y=w343:u32)
        n167 = Wait (ms)(milliseconds to wait=w339) -> ()  [unwired: 1 out]
        n168 = Subtract(x=w342, y=w343) -> (x-y=w338:dbl)
        "Image Acq (s)" <- w338
        n169 = Less Or Equal To 0?(x=w338) -> (x <= 0?=w341:bool)
        n170 = local read "Break"() -> (w336:bool)
        n171 = Or(x=w336, y=w341) -> (x .or. y?=w337:bool)
      }
      n172 = call <vilib>:"DAQmx Stop Task.vi"("task/channels in"=w105, "error in"=w104) -> ("task out"=w103:refnum<k21>, "error out"=w102:errorcluster)  [unwired: 12 in]
      n173 = call <vilib>:"DAQmx Clear Task.vi"("task in"=w103, "error in"=w102) -> ("error out"=w90:errorcluster)  [unwired: 13 in]
      n174 = invoke on="Image Acquisition Started" class="Bool (strict)" method="Reinit To Default"(error in=w90) -> (error out=w89:errorcluster)  [unwired: 2 in, 2 out]
      n175 = disable-structure shown="SCMP==COMP, Default" {
        disable-tunnel: [tag "PXI-6733/port0/line0" ("lines") tag "Dev3/port0/line0" ("comp lines")] -> w57
        disable-tunnel: [tag "PXI-6733/ao0:7" ("physical channels") tag "Dev3/ao0:7" ("physical channels")] -> w56
        frame condition #0 {
        }
        frame condition #1 (active) {
        }
      }
      n176 = call "SCD - Trigger Sequence - Set All AO Values to Zero.vi"("error in"=w89, "lines"=w57, "physical channels"=w56) -> ("error out"=w83:errorcluster)  [unwired: 8 in]
      n177 = Release Queue(queue=w70, error in (no error)=w67) -> (error out=w59:errorcluster)  [unwired: 1 in, 2 out]
      n178 = Merge Errors(w18, w59, w29) -> (w28:errorcluster)
      n179 = Merge Errors(w28, w83) -> (w82:errorcluster)
      "Headers Out" <- w66
      "error dequeue" <- w29
      "Time Start" <- w32
    }
    frame Error {
    }
  }
  "error out" <- w9
  n180 = disable-structure shown="Disabled" {
    frame Disabled {
      # "someday this\nmight speed up\naccumulatons"
      n181 = call "SCD - Extract Image Vector and Timestamp from Pointer.vi"() -> ()  [unwired: 13 in, 3 out]
    }
    frame Enabled {
    }
  }
